vi "Error站_Pause.vi"(8 "error in":errorcluster, 10 "Mode":T1, 11 "ref in":T2) -> (0 "error out":errorcluster, 3 "ref out":T2)   [LabVIEW 2015]
doc: "Use this template to build a VI to use as a subVI."
panel:
  out "Timed out":bool
  in  "ms timeout (-1)":i32=-1
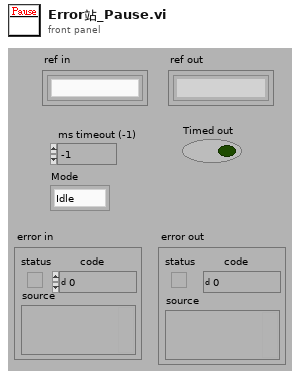
[diagram p1: front panel]
types:
  T1 = typedef "Error站_Mode.ctl" = enum8{"Idle", "Run", "Pause", "Err"}
  T2 = typedef "Error站_ref.ctl" = refnum<k1>
  T3 = enum16{"OpenReference", "CloseReference", "Get Data", "Set Data", "Set Flag"}
  T4 = typedef "Semaphore RefNum" = refnum<k1>
  T5 = typedef "Error站_Data.ctl" = cluster{"GUI":refnum<vi>, "Ready":bool, "Mode":T1, "Function":T6, "Porcedure in":u8, "Time Delay":cluster{"Time Out":dbl, "氣壓缸延遲":dbl, "3":dbl, "4":dbl, "5":dbl, "6":dbl, "7":dbl, "8":dbl, "9":dbl, "10":dbl}, "空跑流程":bool, "異常處理":cluster{"Retry":bool, "Reset":bool, "Skip":bool}, "Message Array":i32[]}
  T6 = typedef "Error站_Function.ctl" = enum8{"預留"}
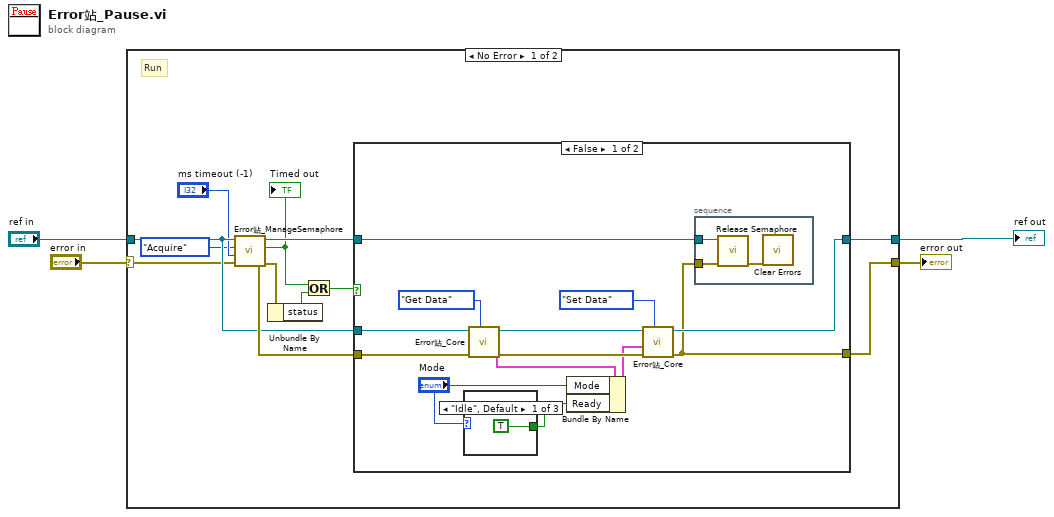
[diagram p0: block diagram]
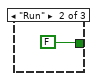
[diagram p2: hidden frame]
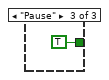
[diagram p3: hidden frame]
diagram:
  n1 = case shown="No Error" "error in" {
    selector: "error in" -> [w6 w38]
    tunnel: [w10 w38] -> w3
    tunnel: "ref in" -> [w11 w37]
    tunnel: [w12 w37] -> w1
    frame No Error {
      # "Run"
      n2 = call "Error站_ManageSemaphore.vi"("error in (no error)"=w6, "ms timeout (-1)"="ms timeout (-1)", "Method (Acquire)"=enum8{"Acquire", "Destroy"}."Acquire", "ref"=w11) -> ("error out"=w15:errorcluster, "Timed out"=w7:bool, "semaphore out"=w13:T4)  [unwired: 1 in]
      "Timed out" <- w7
      n3 = Unbundle By Name(w15) -> ("status"=w8:bool)
      n4 = Or(x=w7, y=w8) -> (x .or. y?=w14:bool)
      n5 = case shown="False" w14 {
        tunnel: [w27 w35] -> w12
        tunnel: w13 -> [w28 _]
        tunnel: w15 -> [w22 w36]
        tunnel: [w26 w36] -> w10
        tunnel: w11 -> [w25 w35]
        frame False {
          n6 = case shown="\"Idle\", Default" "Mode" {
            tunnel: [TRUE ("Ready") FALSE ("Ready") TRUE ("Ready")] -> w23
            frame "Idle", Default {
            }
            frame "Run" {
            }
            frame "Pause" {
            }
          }
          n7 = call "Error站_Core.vi"("Function"=T3."Get Data", "error in"=w22, "ref in"=w25) -> ("error out"=w21:errorcluster, "Data out"=w20:T5, "ref out"=w24:T2)  [unwired: 5 in, 1 out]
          n8 = Bundle By Name(cluster=w20, "Mode"="Mode", "Ready"=w23) -> (w19:T5)
          n9 = call "Error站_Core.vi"("Function"=T3."Set Data", "error in"=w21, "Data in"=w19, "ref in"=w24) -> ("error out"=w26:errorcluster, "ref out"=w27:T2)  [unwired: 4 in, 2 out]
          n10 = stacked-sequence {
            tunnel: w28 -> [w34]
            tunnel: w26 -> [w32]
            frame #0 {
              n11 = call <vilib>:"Release Semaphore.vi"("error in (no error)"=w32, "semaphore"=w34) -> ("error out"=w33:errorcluster)  [unwired: 4 in, 1 out]
              n12 = call <vilib>:"Clear Errors.vi"("error in (no error)"=w33) -> ()  [unwired: 5 in, 2 out]
            }
          }
        }
        frame True {
        }
      }
    }
    frame Error {
    }
  }
  "error out" <- w3
  "ref out" <- w1
